vi "Write Dinero.vi"(8 "error in (no error)":errorcluster, 10 "Dinero":refnum<vi>, 11 "Dinero in":refnum<class "Dinero.lvclass">) -> (0 "error out":errorcluster, 3 "Dinero out":refnum<class "Dinero.lvclass">)   [LabVIEW 2020, in "Dinero.lvlib" / "Dinero.lvclass"]
uses:
  Dinero.lvclass
  Dinero.lvclass/Dinero.ctl
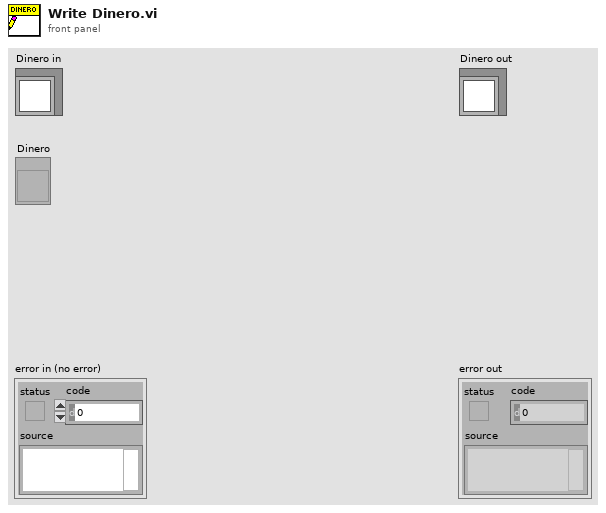
[diagram p1: front panel]
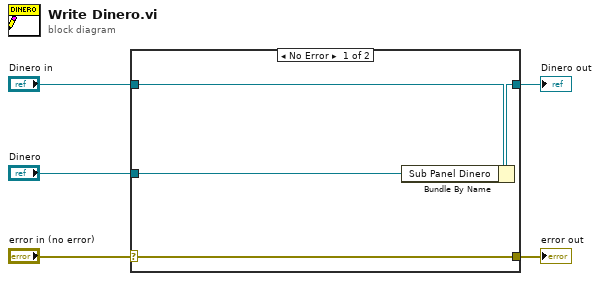
[diagram p0: block diagram]
diagram:
  n1 = case shown="No Error" "error in (no error)" {
    selector: "error in (no error)" -> [w9 w10]
    tunnel: [w9 w10] -> w4
    tunnel: [w7 w11] -> w2
    tunnel: "Dinero in" -> [w8 w11]
    tunnel: "Dinero" -> [w6 _]
    frame No Error {
      n2 = Bundle By Name(cluster=w8, "Sub Panel Dinero"=w6) -> (w7:refnum<class "Dinero.lvclass">)
    }
    frame Error {
    }
  }
  "error out" <- w4
  "Dinero out" <- w2
